vi "Get Step Address(DC Program).vi"(9 "Program Data.Step Number":u32, 10 "Program Data.Mem Number":u32) -> (0 "Program Data.Start Address (Low)":string, 1 "Program Data.Start Address (Middle Low)":string, 2 "Program Data.Start Address (Middle High)":string, 3 "Program Data.Start Address (High)":string, 5 "Length (Low)":string, 7 "Length (High)":string)   [LabVIEW 2013]
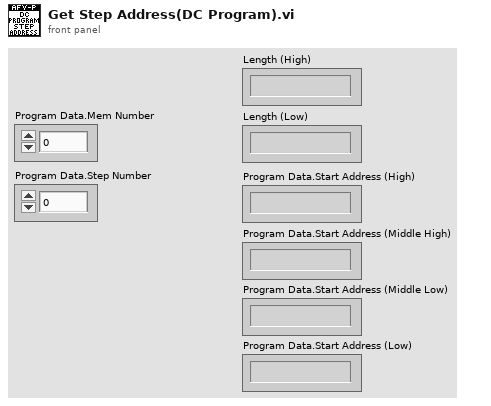
[diagram p1: front panel]
types:
  T1 = cluster{"Start Address (High)":string, "Start Address (Middle High)":string, "Start Address (Middle Low)":string, "Start Address (Low)":string, "Step Length":string, "Mem Number":u32, "Step Number":u32}
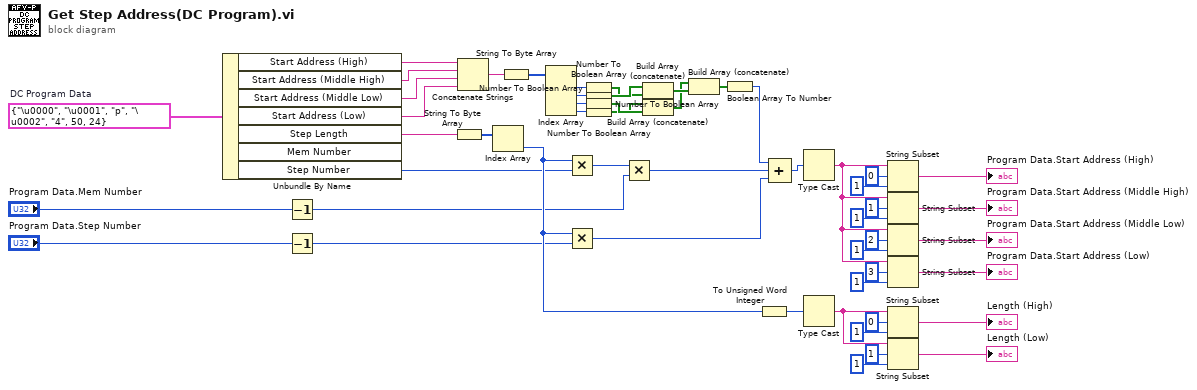
[diagram p0: block diagram]
diagram:
  w5 = T1 {"Start Address (High)"="\u0000", "Start Address (Middle High)"="\u0001", "Start Address (Middle Low)"="p", "Start Address (Low)"="\u0002", "Step Length"="4", "Mem Number"=50, "Step Number"=24}  # DC Program Data
  n1 = Unbundle By Name(w5) -> ("Start Address (High)"=w11:string, "Start Address (Middle High)"=w10:string, "Start Address (Middle Low)"=w9:string, "Start Address (Low)"=w8:string, "Step Length"=w7:string, "Step Number"=w6:u32)  [unwired: 1 out]
  n2 = Decrement(x="Program Data.Mem Number") -> (x-1=w3:u32)
  n3 = Decrement(x="Program Data.Step Number") -> (x-1=w1:u32)
  n4 = String To Byte Array(string=w7) -> (unsigned byte array=w33:u8[])
  n5 = Concatenate Strings(w11, w10, w9, w8) -> (w43:string)
  n6 = Index Array(array=w33) -> (element=w12:u8)  [unwired: 1 in]
  n7 = String To Byte Array(string=w43) -> (unsigned byte array=w46:u8[])
  n8 = Index Array(array=w46) -> (element #1=w40:u8, element #2=w39:u8, element #3=w45:u8, element #4=w44:u8)  [unwired: 4 in]
  n9 = Multiply(x=w12, y=w6) -> (x*y=w15:u32)
  n10 = Multiply(x=w12, y=w1) -> (x*y=w13:u32)
  n11 = Number To Boolean Array(number=w40) -> (Boolean array=w37:bool[])
  n12 = Number To Boolean Array(number=w39) -> (Boolean array=w38:bool[])
  n13 = Number To Boolean Array(number=w45) -> (Boolean array=w42:bool[])
  n14 = Number To Boolean Array(number=w44) -> (Boolean array=w41:bool[])
  n15 = Multiply(x=w15, y=w3) -> (x*y=w21:u32)
  n16 = Build Array (concatenate)(w38, w37) -> (w36:bool[])
  n17 = Build Array (concatenate)(w41, w42) -> (w35:bool[])
  n18 = Build Array (concatenate)(w35, w36) -> (w34:bool[])
  n19 = Boolean Array To Number(Boolean array=w34) -> (number=w32:u32)
  n20 = To Unsigned Word Integer(number=w12) -> (unsigned 16bit integer=w14:u16)
  n21 = Compound Arithmetic op=ADD(w32, w21, w13) -> (w22:u32)
  n22 = Type Cast(x=w22) -> (*(type *) &x=w23:string)  [unwired: 1 out]
  n23 = Type Cast(x=w14) -> (*(type *) &x=w16:string)  [unwired: 1 out]
  n24 = String Subset(string=w23, offset (0)=0, length (rest)=1 ("length (rest)")) -> (substring=→"Program Data.Start Address (High)":string)
  n25 = String Subset(string=w23, offset (0)=1, length (rest)=1 ("length (rest)")) -> (substring=→"Program Data.Start Address (Middle High)":string)
  n26 = String Subset(string=w23, offset (0)=2, length (rest)=1 ("length (rest)")) -> (substring=→"Program Data.Start Address (Middle Low)":string)
  n27 = String Subset(string=w23, offset (0)=3, length (rest)=1 ("length (rest)")) -> (substring=→"Program Data.Start Address (Low)":string)
  n28 = String Subset(string=w16, offset (0)=0, length (rest)=1 ("length (rest)")) -> (substring=→"Length (High)":string)
  n29 = String Subset(string=w16, offset (0)=1, length (rest)=1 ("length (rest)")) -> (substring=→"Length (Low)":string)
